vi "Weight sensor and Gas Sensor.vi"() -> ()   [LabVIEW 2022 SP3]
uses:
  <vilib>/DAQmx/miscellaneous.llb/DAQmx Fill In Error Info.vi
  <vilib>/DAQmx/create/channels.llb/DAQmx Create Channel (DO-Digital Output).vi
  <vilib>/DAQmx/write.llb/DAQmx Write (Digital Bool 1Line 1Point).vi
  <vilib>/DAQmx/read.llb/DAQmx Read (Analog 1D DBL NChan 1Samp).vi
  <vilib>/DAQmx/create/channels.llb/DAQmx Create Channel (AI-Voltage-Basic).vi
panel:
  out "Square 2":dynamicdata(graph) caption="Square"
  in  "Frequency 3":dbl=50.0 caption="Frequency"
  in  "Offset 3":dbl=2.5 caption="Offset"
  in  "Amplitude 3":dbl=2.5 caption="Amplitude"
  out "Square":dynamicdata(graph)
  in  "Frequency":dbl=50.0
  in  "Offset":dbl=2.5
  in  "Amplitude":dbl=2.5
  out "gas analog read value":dbl
  in  "buzzer output channel":tag
  out "Boolean":bool
  out "gas detection":dbl(knob) scale=0.0..10.0
  out "Weight":dbl(knob) scale=0.0..800.0
  out "Weight":dbl
  out "Voltage":dbl format="%0.2f"
  in  "physical channels- weight sensor/ gas sensor":tag
  in  "stop":bool
  # "GAS SENSOR"
  # "WEIGHT SENSOR"
  # "SERVO MOTOR"
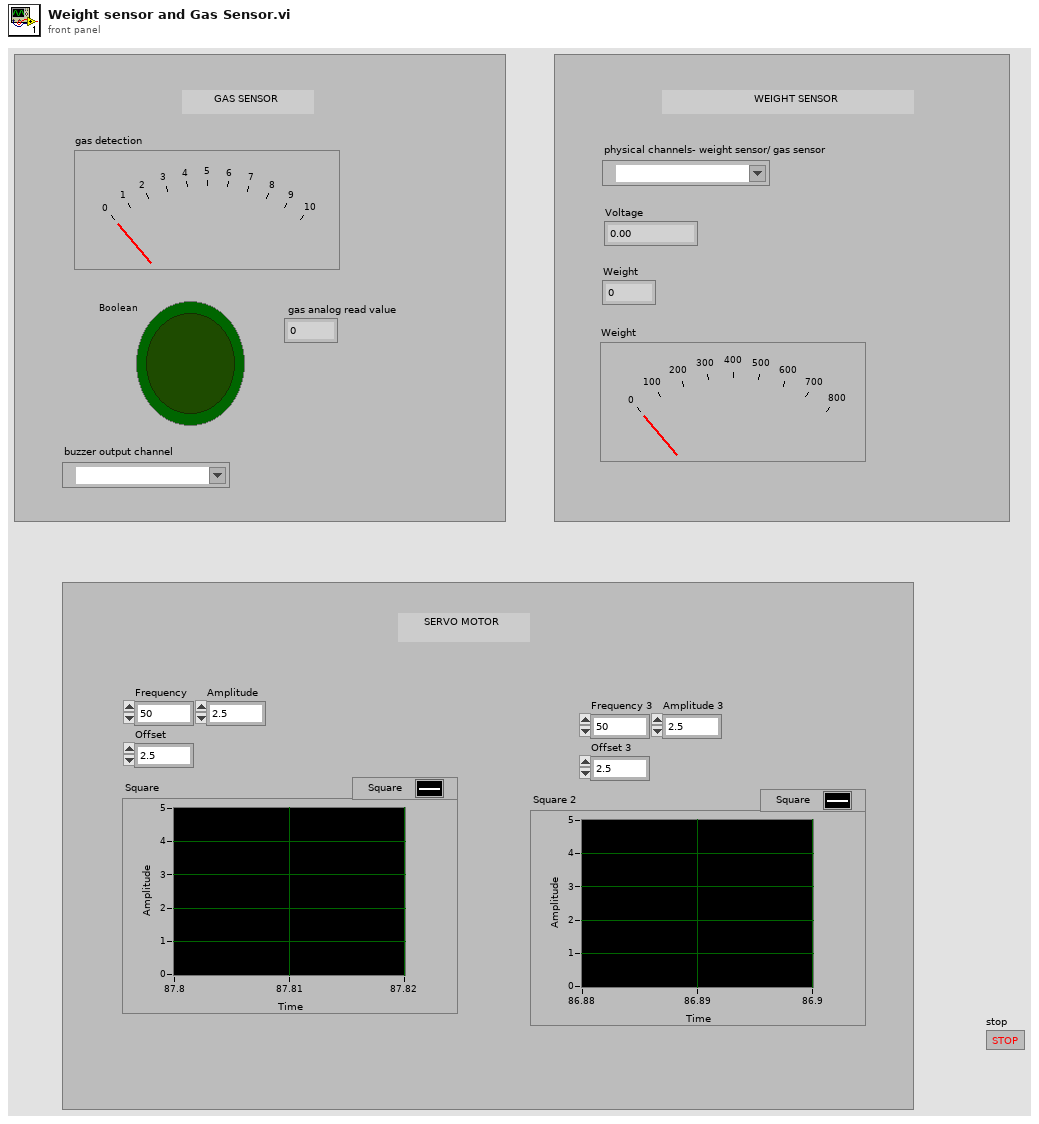
[diagram p1: front panel]
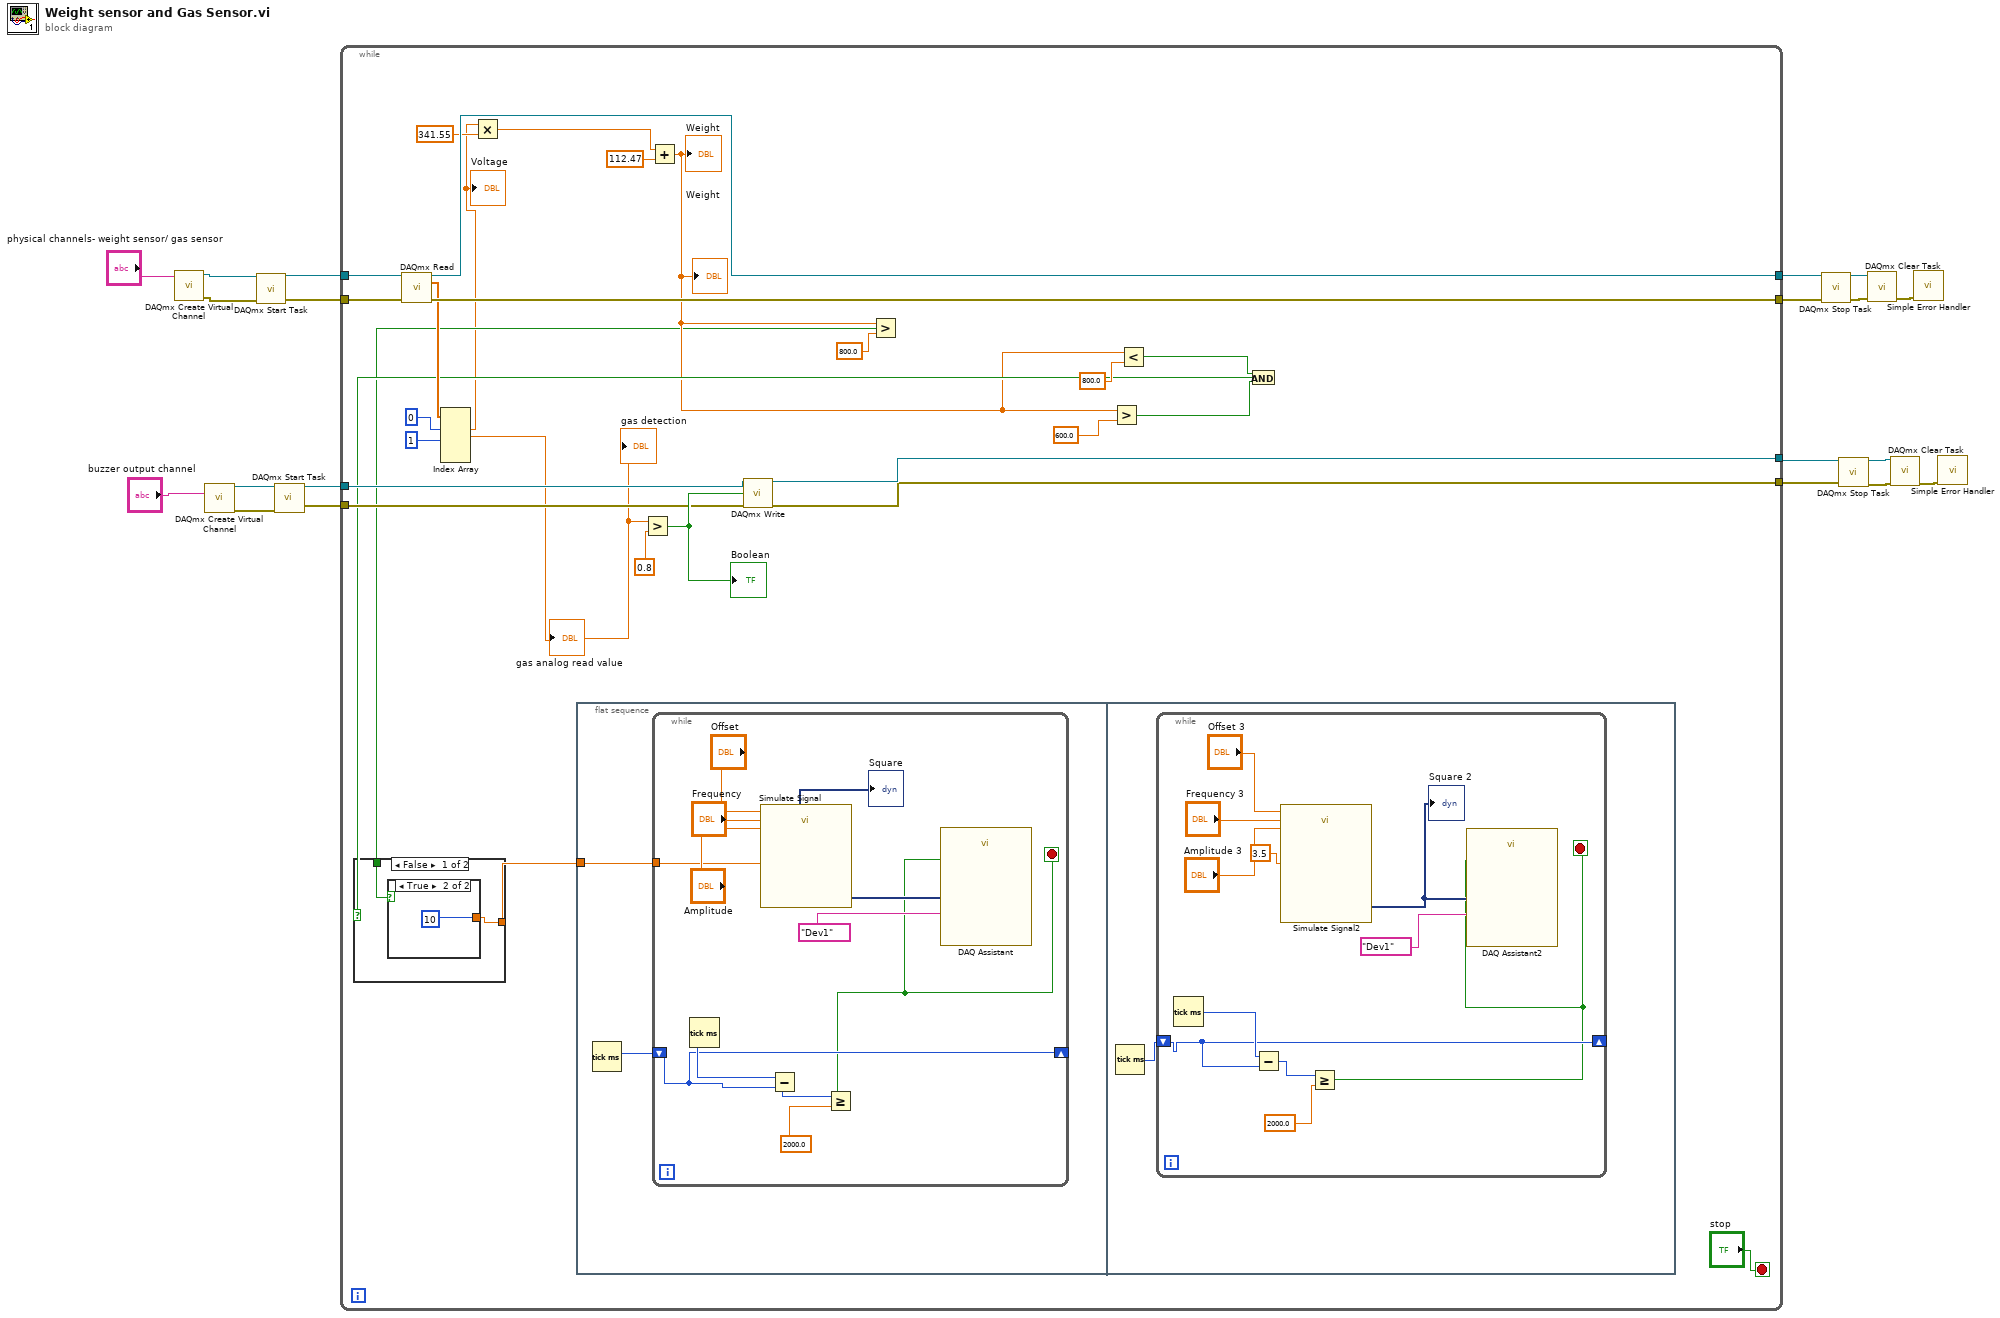
[diagram p0: block diagram]
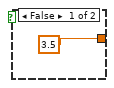
[diagram p2: hidden frame]
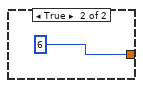
[diagram p3: hidden frame]
diagram:
  n1 = call-poly <vilib>:"DAQmx Create Virtual Channel.vi"("physical channels"="physical channels- weight sensor/ gas sensor") -> ("task out"=w20:refnum<k21>, "error out"=w19:errorcluster)  [unwired: 13 in]
  n2 = call-poly <vilib>:"DAQmx Create Virtual Channel.vi"("lines"="buzzer output channel") -> ("task out"=w10:refnum<k21>, "error out"=w9:errorcluster)  [unwired: 13 in]
  n3 = call <vilib>:"DAQmx Start Task.vi"("task/channels in"=w20, "error in"=w19) -> ("task out"=w18:refnum<k21>, "error out"=w17:errorcluster)  [unwired: 12 in]
  n4 = call <vilib>:"DAQmx Start Task.vi"("task/channels in"=w10, "error in"=w9) -> ("task out"=w3:refnum<k21>, "error out"=w2:errorcluster)  [unwired: 12 in]
  n5 = while {
    tunnel: w18 -> [w48]
    tunnel: w17 -> [w47]
    tunnel: [w46] -> w16
    tunnel: [w45] -> w13
    tunnel: [w36] -> w6
    tunnel: [w35] -> w5
    tunnel: w3 -> [w34]
    tunnel: w2 -> [w33]
    stop <- "stop" stop-if-true
    n6 = call-poly <vilib>:"DAQmx Read.vi"("task/channels in"=w48, "error in"=w47) -> ("task out"=w46:refnum<k21>, "data"=w41:dbl[], "error out"=w45:errorcluster)  [unwired: 11 in]
    n7 = Index Array(array=w41, index #1=0 ("index"), index #2=1 ("index")) -> (element #1=w22:dbl, element #2=w31:dbl)  [unwired: 3 in, 3 out]
    "Voltage" <- w22
    "gas analog read value" <- w31
    "gas detection" <- w31
    n8 = Multiply(x=w22, y=341.55) -> (x*y=w21:dbl)
    n9 = flat-sequence {
      tunnel: w30 -> [w49]
      frame #0 {
        n10 = Tick Count (ms)() -> (millisecond timer value=w50:u32)
        n11 = while {
          shift-right: [w53] -> _
          shift-left: w50 -> [w53]
          tunnel: w49 -> [w51]
          stop <- w52 stop-if-true
          n12 = Tick Count (ms)() -> (millisecond timer value=w55:u32)
          n13 = call "Simulate Signal"("Offset"="Offset", "Duty Cycle (%)"=w51, "Frequency"="Frequency", "Amplitude"="Amplitude") -> ("Square"=w58:dynamicdata)  [unwired: 10 in, 1 out]
          "Square" <- w58
          n14 = Subtract(x=w55, y=w53) -> (x-y=w54:u32)
          n15 = Greater Or Equal?(x=w54, y=2000.0 ("Time Target (s)")) -> (x >= y?=w52:bool)
          n16 = call "DAQ Assistant"("data"=w58, "stop (F)"=w52, "device name"=tag "Dev1") -> ()  [unwired: 14 in, 3 out]
        }
      }
      frame #1 {
        n17 = Tick Count (ms)() -> (millisecond timer value=w62:u32)
        n18 = while {
          shift-right: [w64] -> _
          shift-left: w62 -> [w64]
          stop <- w63 stop-if-true
          n19 = Tick Count (ms)() -> (millisecond timer value=w66:u32)
          n20 = Subtract(x=w66, y=w64) -> (x-y=w65:u32)
          n21 = call "Simulate Signal2"("Offset"="Offset 3", "Duty Cycle (%)"=3.5, "Frequency"="Frequency 3", "Amplitude"="Amplitude 3") -> ("Square"=w70:dynamicdata)  [unwired: 10 in, 1 out]
          "Square 2" <- w70
          n22 = Greater Or Equal?(x=w65, y=2000.0 ("Time Target (s)")) -> (x >= y?=w63:bool)
          n23 = call "DAQ Assistant2"("data"=w70, "stop (F)"=w63, "device name"=tag "Dev1") -> ()  [unwired: 14 in, 3 out]
        }
      }
    }
    n24 = Greater?(x=w31, y=0.8) -> (0:w37:bool)
    "Boolean" <- w37
    n25 = Add(x=w21, y=112.47) -> (x+y=w24:dbl)
    "Weight" <- w24
    "Weight" <- w24
    n26 = call-poly <vilib>:"DAQmx Write.vi"("task/channels in"=w34, "data"=w37, "error in"=w33) -> ("task out"=w36:refnum<k21>, "error out"=w35:errorcluster)  [unwired: 10 in, 1 out]
    n27 = Greater?(x=w24, y=800.0) -> (0:w23:bool)
    n28 = Greater?(x=w24, y=600.0) -> (0:w27:bool)
    n29 = Less?(x=w24, y=800.0) -> (x < y?=w28:bool)
    n30 = And(x=w28, y=w27) -> (x .and. y?=w26:bool)
    n31 = case shown="False" w26 {
      tunnel: [w74 6] -> w30
      tunnel: w23 -> [w75 _]
      frame False {
        n32 = case shown="True" w75 {
          tunnel: [3.5 10] -> w74
          frame False {
          }
          frame True {
          }
        }
      }
      frame True {
      }
    }
  }
  n33 = call <vilib>:"DAQmx Stop Task.vi"("task/channels in"=w16, "error in"=w13) -> ("task out"=w15:refnum<k21>, "error out"=w1:errorcluster)  [unwired: 12 in]
  n34 = call <vilib>:"DAQmx Stop Task.vi"("task/channels in"=w6, "error in"=w5) -> ("task out"=w7:refnum<k21>, "error out"=w4:errorcluster)  [unwired: 12 in]
  n35 = call <vilib>:"DAQmx Clear Task.vi"("task in"=w15, "error in"=w1) -> ("error out"=w14:errorcluster)  [unwired: 13 in]
  n36 = call <vilib>:"DAQmx Clear Task.vi"("task in"=w7, "error in"=w4) -> ("error out"=w8:errorcluster)  [unwired: 13 in]
  n37 = call <vilib>:"Simple Error Handler.vi"("error in (no error)"=w14) -> ()  [unwired: 4 in, 5 out]
  n38 = call <vilib>:"Simple Error Handler.vi"("error in (no error)"=w8) -> ()  [unwired: 4 in, 5 out]
